vi "failure1.vi"() -> ()   [LabVIEW 2018]
panel:
  in  "stop":bool
  out "current time 2":timestamp
  in  "current time":timestamp
  in  "Numeric 2":dbl
  in  "Numeric":dbl
  in  "String":string
  in  "Table":string[][](table)
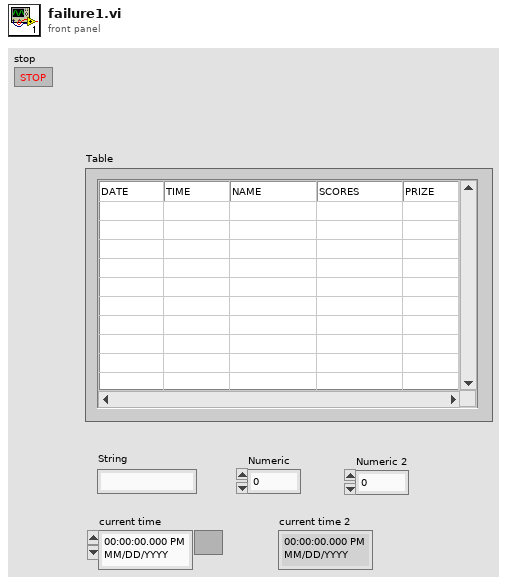
[diagram p1: front panel]
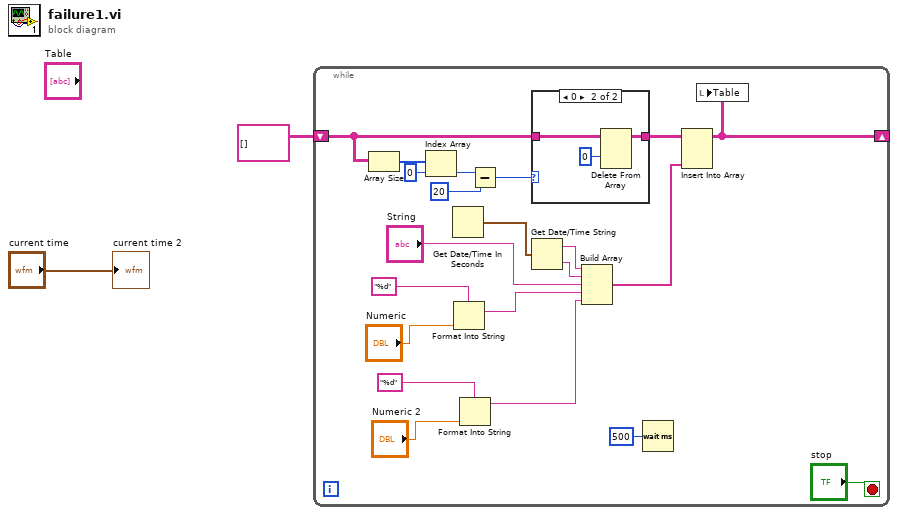
[diagram p0: block diagram]
diagram:
  n1 = while {
    shift-right: [w23] -> _
    shift-left: string[][] [] -> [w17]
    stop <- "stop" stop-if-true
    n2 = Array Size(array=w17) -> (size(s)=w16:i32[])
    n3 = Index Array(array=w16, index=0) -> (element=w14:i32)
    n4 = Get Date/Time In Seconds() -> (seconds since 1Jan1904=w4:timestamp)
    n5 = Format Into String(format string="%d" ("initial string"), "Numeric") -> (resulting string=w9:string)  [unwired: 2 in, 1 out]
    n6 = Format Into String(format string="%d" ("initial string"), "Numeric 2") -> (resulting string=w5:string)  [unwired: 2 in, 1 out]
    n7 = Subtract(x=w14, y=20) -> (x-y=w13:i32)
    n8 = case shown="0" w13 {
      tunnel: w17 -> [w24 w27]
      tunnel: [w24 w26] -> w18
      frame Default {
      }
      frame 0 {
        n9 = Delete From Array(array=w27, index (row)=0) -> (array with subset deleted=w26:string[][])  [unwired: 2 in, 1 out]
      }
    }
    n10 = Get Date/Time String(seconds (now)=w4) -> (date string=w21:string, time string=w22:string)  [unwired: 2 in]
    n11 = Build Array(w21, w22, "String", w9, w5) -> (w20:string[])
    n12 = Wait (ms)(milliseconds to wait=u32 500) -> ()  [unwired: 1 out]
    n13 = Insert Into Array(array=w18, new element=w20) -> (w23:string[][])  [unwired: 2 in]
    n14 = local write "Table"(w23) -> ()
  }
  "current time 2" <- "current time"
